vi "Log Message.vi"(8 "error in (no error)":errorcluster, 10 "Message":string, 11 "CoolAppProcess in":refnum<class "CoolAppProcess.lvclass">) -> (0 "error out":errorcluster, 3 "CoolAppProcess out":refnum<class "CoolAppProcess.lvclass">)   [LabVIEW 2020, in "LAF2024Q2.lvlib" / "CoolAppProcess.lvclass"]
uses:
  CoolAppProcess.lvclass
  CoolAppProcess.lvclass/CoolAppProcess.ctl
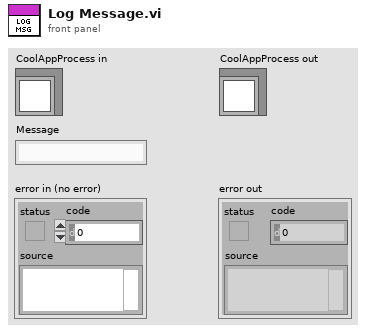
[diagram p1: front panel]
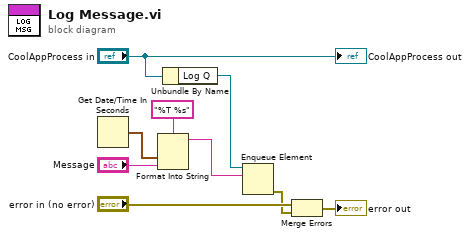
[diagram p0: block diagram]
diagram:
  n1 = Get Date/Time In Seconds() -> (seconds since 1Jan1904=w8:timestamp)
  n2 = Format Into String(format string="%T %s", w8, "Message") -> (resulting string=w4:string)  [unwired: 2 in, 1 out]
  n3 = Unbundle By Name("CoolAppProcess in") -> ("Log Q"=w5:refnum<queue>)
  n4 = Enqueue Element(queue=w5, element=w4) -> (error out=w2:errorcluster)  [unwired: 2 in, 2 out]
  n5 = Merge Errors("error in (no error)", w2) -> (→"error out":errorcluster)
  "CoolAppProcess out" <- "CoolAppProcess in"
